vi "Init Rx - Data.vi"(7 "Data Access in":refnum<class "Data Access Engine.lvclass">, 8 "error in (no error)":errorcluster, 11 "Parameters":variant) -> (0 "error out":errorcluster, 3 "Rx Loop Data":T1, 5 "Data Access out":refnum<class "Data Access Engine.lvclass">)   [LabVIEW 2016, in "UDP-Custom-Device Engine.lvlib"]
uses:
  UDP-Custom-Device Engine.lvlib
  Types/Engine - Rx Loop Data.ctl
  <vilib>/NI Veristand/VeriStand Data/Library/Byte Buffer/Byte Buffer.lvclass
  <vilib>/NI/NIVS Inline Async API/_Data Access Engine/Data Access Engine/Types/Write.DVR.ctl
  <vilib>/NI/NIVS Inline Async API/_Data Access Engine/Access Type Classes/Write/Write.lvclass
  <vilib>/NI Veristand/VeriStand Data/Library/Typedefs/Typedefs.Data Types.ctl
  Types/Engine - Data Conversion Config.ctl
  <vilib>/NI Veristand/VeriStand Data/Library/Byte Buffer/Byte Buffer.Mapping.ctl
  Shared/Types/Shared - Header Details.ctl
  Shared/Types/Shared - Duplex Settings.ctl
  <vilib>/NI/NIVS Inline Async API/_Data Access Engine/Data Access Engine/Data Access Engine.lvclass
  Shared/Types/Shared - Rx.PacketInfo.ctl
  Shared/Types/Shared - Channel Data Type.ctl
  Shared/Types/Shared - Buffered.PacketInfo.ctl
  <vilib>/NI/NIVS Inline Async API/_Data Access Engine/Data Access Engine/Methods/Write.Lookup.vi
  Shared/UDP-Custom-Device Shared.lvlib
  <vilib>/NI Veristand/VeriStand Data/Library/VeriStand Data.lvlib
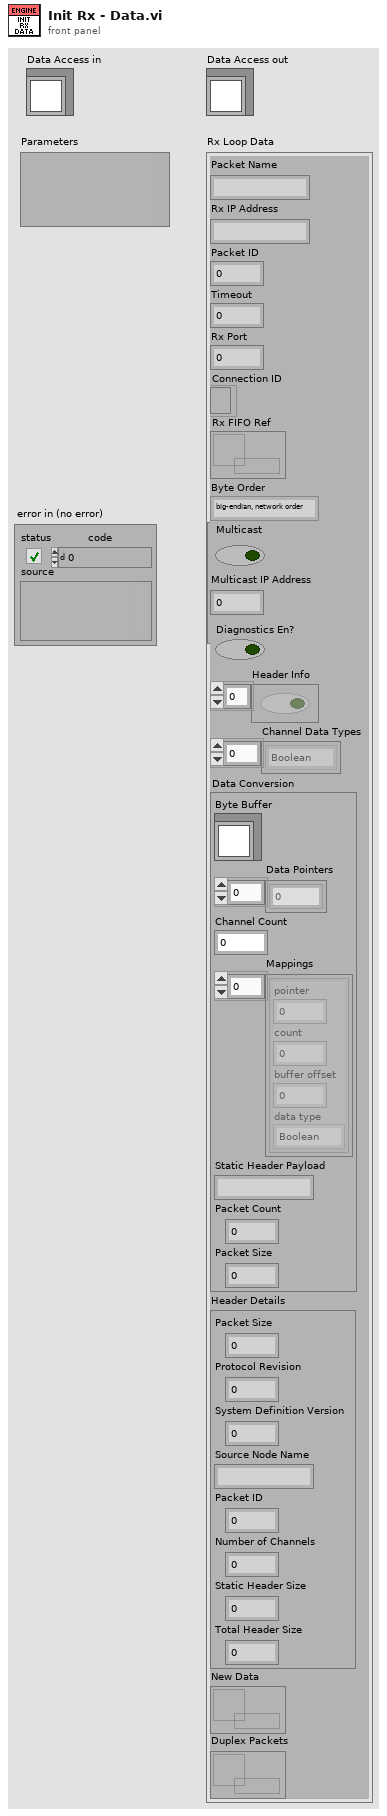
[diagram p1: front panel]
types:
  T1 = typedef "UDP-Custom-Device Engine.lvlib/Engine - Rx Loop Data.ctl" = cluster{"Packet Name":string, "Rx IP Address":string, "Packet ID":i32, "Timeout":i32, "Rx Port":i32, "Connection ID":refnum<k16>, "Rx FIFO Ref":T2, "Byte Order":enum16{"big-endian, network order", "native, host order", "little-endian"}, "Multicast":bool, "Multicast IP Address":u32, "Diagnostics En?":bool, "Header Info":bool[], "Channel Data Types":T3[], "Data Conversion":T4, "Header Details":T6, "New Data":T2, "Duplex Packets":refnum<data-value>}
  T2 = typedef "Data Access Engine.lvlib/Data Access Engine.lvclass/Write.DVR.ctl" = refnum<data-value>
  T3 = typedef "VeriStand Data.lvlib/Typedefs.Data Types.ctl" = enum16{"Boolean", "Single", "Double", "I8", "I16", "I32", "I64", "U8", "U16", "U32", "U64"}
  T4 = typedef "UDP-Custom-Device Engine.lvlib/Engine - Data Conversion Config.ctl" = cluster{"Byte Buffer":refnum<class "Byte Buffer.lvclass">, "Data Pointers":u64[], "Channel Count":i32, "Mappings":T5[], "Static Header Payload":string, "Packet Count":dbl, "Packet Size":i32}
  T5 = typedef "VeriStand Data.lvlib/Byte Buffer.lvclass/Byte Buffer.Mapping.ctl" = cluster{"pointer":u64, "count":i32, "buffer offset":i32, "data type":T3}
  T6 = typedef "UDP-Custom-Device Shared.lvlib/Shared - Header Details.ctl" = cluster{"Packet Size":u16, "Protocol Revision":u8, "System Definition Version":u64, "Source Node Name":string, "Packet ID":u32, "Number of Channels":u32, "Static Header Size":u16, "Total Header Size":u16}
  T7 = typedef "UDP-Custom-Device Shared.lvlib/Shared - Rx.PacketInfo.ctl" = cluster{"Packet Name":string, "Packet ID":i32, "Timeout":i32, "Rx IP Address":string, "Rx Port":u16, "Endianness":u16, "Multicast":bool, "Multicast IP Address":string, "Diagnostics En?":bool, "Header Info":bool[], "Channel Data Types":T8[], "Buffered Packet Info":T9, "Duplex Packets":refnum<data-value>}
  T8 = typedef "UDP-Custom-Device Shared.lvlib/Shared - Channel Data Type.ctl" = enum16{"Boolean", "Single", "Double", "I8", "I16", "I32", "I64", "U8", "U16", "U32", "U64"}
  T9 = typedef "UDP-Custom-Device Shared.lvlib/Shared - Buffered.PacketInfo.ctl" = cluster{"Buffer Size":i32, "External Buffer":bool, "Prepend Header":bool, "Is Buffered":bool}
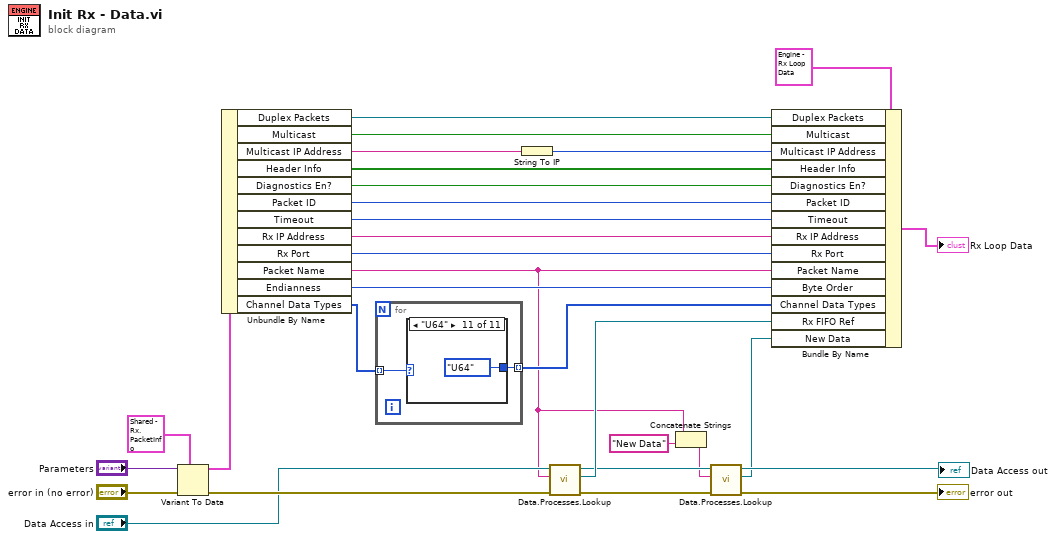
[diagram p0: block diagram]
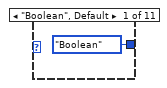
[diagram p2: hidden frame]
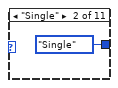
[diagram p3: hidden frame]
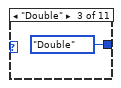
[diagram p4: hidden frame]
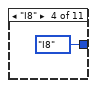
[diagram p5: hidden frame]
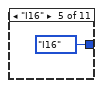
[diagram p6: hidden frame]
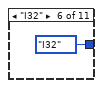
[diagram p7: hidden frame]
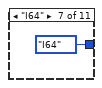
[diagram p8: hidden frame]
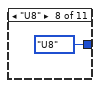
[diagram p9: hidden frame]
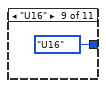
[diagram p10: hidden frame]
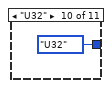
[diagram p11: hidden frame]
diagram:
  n1 = Variant To Data(error in="error in (no error)", type=T7 {"Packet Name"="", "Packet ID"=0, "Timeout"=0, "Rx IP Address"="", "Rx Port"=0, "Endianness"=0, "Multicast"=FALSE, "Multicast IP Address"="", "Diagnostics En?"=FALSE, "Header Info"=[], "Channel Data Types"=[], "Buffered Packet Info"={"Buffer Size"=0, "External Buffer"=FALSE, "Prepend Header"=FALSE, "Is Buffered"=FALSE}, "Duplex Packets"=refnum} ("Packet Info"), Variant="Parameters") -> (data=w27:T7, error out=w20:errorcluster)
  n2 = Unbundle By Name(w27) -> ("Duplex Packets"=w1:refnum<data-value>, "Multicast"=w4:bool, "Multicast IP Address"=w3:string, "Header Info"=w15:bool[], "Diagnostics En?"=w16:bool, "Packet ID"=w21:i32, "Timeout"=w22:i32, "Rx IP Address"=w23:string, "Rx Port"=w24:u16, "Packet Name"=w6:string, "Endianness"=w17:u16, "Channel Data Types"=w14:T8[])
  n3 = for {
    tunnel: w14 -> [w32] mode=indexing
    tunnel: [w31] -> w13 mode=indexing
    n4 = case shown="\"U64\"" w32 {
      tunnel: [Typedefs.Data_Types."Boolean" ("data type") Typedefs.Data_Types."Single" ("data type") Typedefs.Data_Types."Double" ("data type") Typedefs.Data_Types."I8" ("data type") Typedefs.Data_Types."I16" ("data type") Typedefs.Data_Types."I32" ("data type") Typedefs.Data_Types."I64" ("data type") Typedefs.Data_Types."U8" ("data type") Typedefs.Data_Types."U16" ("data type") Typedefs.Data_Types."U32" ("data type") Typedefs.Data_Types."U64" ("data type")] -> w31
      frame "Boolean", Default {
      }
      frame "Single" {
      }
      frame "Double" {
      }
      frame "I8" {
      }
      frame "I16" {
      }
      frame "I32" {
      }
      frame "I64" {
      }
      frame "U8" {
      }
      frame "U16" {
      }
      frame "U32" {
      }
      frame "U64" {
      }
    }
  }
  n5 = String To IP(1:w3) -> (0:w2:u32)
  n6 = call-poly <vilib>:"Data.Processes.Lookup.vi"("error in (no error)"=w20, "Name"=w6, "Data Access API in"="Data Access in") -> ("error out"=w10:errorcluster, "Ref"=w18:T2, "Data Access API out"=w12:refnum<class "Data Access Engine.lvclass">)  [unwired: 5 in, 1 out]
  n7 = Concatenate Strings(w6, "New Data" ("Item GUID")) -> (w5:string)
  n8 = call-poly <vilib>:"Data.Processes.Lookup.vi"("error in (no error)"=w10, "Name"=w5, "Data Access API in"=w12) -> ("error out"=→"error out":errorcluster, "Ref"=w8:T2, "Data Access API out"=→"Data Access out":refnum<class "Data Access Engine.lvclass">)  [unwired: 5 in, 1 out]
  n9 = Bundle By Name(cluster=T1 {"Packet Name"="", "Rx IP Address"="", "Packet ID"=0, "Timeout"=0, "Rx Port"=0, "Connection ID"=refnum, "Rx FIFO Ref"=refnum, "Byte Order"=enum."big-endian, network order", "Multicast"=FALSE, "Multicast IP Address"=0, "Diagnostics En?"=FALSE, "Header Info"=[], "Channel Data Types"=[], "Data Conversion"={"Byte Buffer"=refnum, "Data Pointers"=[], "Channel Count"=0, "Mappings"=[], "Static Header Payload"="", "Packet Count"=0.0, "Packet Size"=0}, "Header Details"={"Packet Size"=0, "Protocol Revision"=0, "System Definition Version"=0, "Source Node Name"="", "Packet ID"=0, "Number of Channels"=0, "Static Header Size"=0, "Total Header Size"=0}, "New Data"=refnum, "Duplex Packets"=refnum} ("Rx Loop Data"), "Duplex Packets"=w1, "Multicast"=w4, "Multicast IP Address"=w2, "Header Info"=w15, "Diagnostics En?"=w16, "Packet ID"=w21, "Timeout"=w22, "Rx IP Address"=w23, "Rx Port"=w24, "Packet Name"=w6, "Byte Order"=w17, "Channel Data Types"=w13, "Rx FIFO Ref"=w18, "New Data"=w8) -> (→"Rx Loop Data":T1)
